vi "Program Setup.vi"(8 "error in (no error)":errorcluster, 10 "shutdown":refnum<user-event>, 11 "Modules":T8) -> (0 "error out":errorcluster)   [LabVIEW 2025]
uses:
  Controls/Sequencer/save icon.ctl
  Controls/transparent tab control.ctl
  Controls/refresh button 2.ctl
  Controls/tests tab control.ctl
  Controls/json cluster.ctl
  <vilib>/Handler Framework/CmdQueue/Enqueue Single.vi
  00f64e30-74e4-4e09-a3ad-345c80b98643.vi
  <vilib>/JDP Science/JSONtext/Variant to JSON Text.vi
  <vilib>/JDP Science/JSONtext/LVClass Serializer/JSONtext LVClass Serializer.lvclass
  <vilib>/Handler Framework/Handler Framework.lvlib
  <vilib>/JDP Science/JSONtext/JSONtext.lvlib
  aee85382-6405-4b67-82e5-8524274b1efe.vi
panel:
  in  "Tab Control":T1
  in  "Program":u16(ring) items=["AC-97", "EVI-79"]
  in  "Refresh":T2
  in  "Tab Control 3":T3
  out "Wear_in 2":T4={"V"=24.0, "I"=0.5, "Cycles"=50.0, "On_Time_ms"=100.0, "Off_Time_ms"=900.0}
  out "Drop_out 2":T5={"V"=24.0, "I"=0.5, "V_reduced"=4.0, "V_perturb"=0.01, "Plunger_Threshold"=0.01, "V_MIN"=1.0}
  out "CRT 2":cluster{"V":dbl, "I":dbl, "CRT_MAX_ms":dbl}={"V"=24.0, "I"=0.5, "CRT_MAX_ms"=100.0}
  out "Pull_in 2":T6={"V"=0.0, "I"=0.5, "V_increased"=9.0, "V_perturb"=0.01, "Plunger_Threshold"=0.01, "V_MAX"=13.0}
  out "Electrical_Properties 2":cluster{"V_max":dbl, "I_max":dbl}={"V_max"=24.0, "I_max"=0.5}
  out "ORT 2":cluster{"V":dbl, "I":dbl, "ORT_MAX_ms":dbl}={"V"=24.0, "I"=0.5, "ORT_MAX_ms"=100.0}
  in  "Program Name":string
  in  "Tab Control 2":T3
  in  "Wear_in":T4={"V"=24.0, "I"=0.5, "Cycles"=50.0, "On_Time_ms"=100.0, "Off_Time_ms"=900.0}
  in  "Drop_out":T5={"V"=24.0, "I"=0.5, "V_reduced"=4.0, "V_perturb"=0.01, "Plunger_Threshold"=0.01, "V_MIN"=1.0}
  in  "CRT":cluster{"V":dbl, "I":dbl, "CRT_MAX_ms":dbl}={"V"=24.0, "I"=0.5, "CRT_MAX_ms"=100.0}
  in  "Pull_in":T6={"V"=0.0, "I"=0.5, "V_increased"=9.0, "V_perturb"=0.01, "Plunger_Threshold"=0.01, "V_MAX"=13.0}
  in  "Electrical_Properties":cluster{"V_max":dbl, "I_max":dbl}={"V_max"=24.0, "I_max"=0.5}
  in  "ORT":cluster{"V":dbl, "I":dbl, "ORT_MAX_ms":dbl}={"V"=24.0, "I"=0.5, "ORT_MAX_ms"=100.0}
  in  "Save Program":T7
  # "Edit Programs"
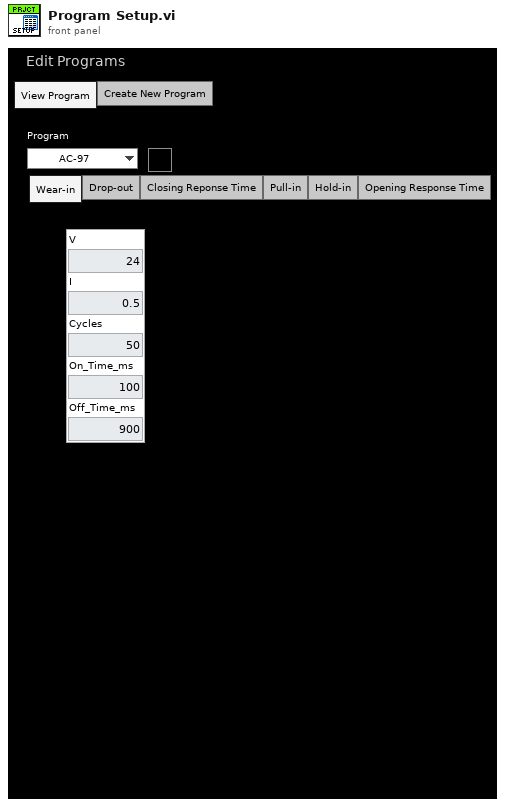
[diagram p1: front panel]
types:
  T1 = typedef "transparent tab control.ctl" = enum32{"View Program", "Create New Program"}
  T2 = typedef "refresh button 2.ctl" = bool
  T3 = typedef "tests tab control.ctl" = enum32{"Wear-in", "Drop-out", "Closing Reponse Time", "Pull-in", "Hold-in", "Opening Response Time"}
  T4 = cluster{"V":dbl, "I":dbl, "Cycles":dbl, "On_Time_ms":dbl, "Off_Time_ms":dbl}
  T5 = cluster{"V":dbl, "I":dbl, "V_reduced":dbl, "V_perturb":dbl, "Plunger_Threshold":dbl, "V_MIN":dbl}
  T6 = cluster{"V":dbl, "I":dbl, "V_increased":dbl, "V_perturb":dbl, "Plunger_Threshold":dbl, "V_MAX":dbl}
  T7 = typedef "save icon.ctl" = bool
  T8 = cluster{"Module IDs":i32[], "Module Names":string[]}
  T9 = enum16{"open", "replace", "create", "open or create", "replace or create", "replace or create with confirmation"}
  T10 = typedef "json cluster.ctl" = cluster{"Electrical_Properties":cluster{"V_max":dbl, "I_max":dbl}, "Wear_in":cluster{"V":dbl, "I":dbl, "Cycles":dbl, "On_Time_ms":dbl, "Off_Time_ms":dbl}, "Drop_out":cluster{"V":dbl, "I":dbl, "V_reduced":dbl, "V_perturb":dbl, "Plunger_Threshold":dbl, "V_MIN":dbl}, "ORT":cluster{"V":dbl, "I":dbl, "ORT_MAX_ms":dbl}, "CRT":cluster{"V":dbl, "I":dbl, "ORT_MAX_ms":dbl}, "Pull_in":cluster{"V":dbl, "I":dbl, "V_increased":dbl, "V_perturb":dbl, "Plunger_Threshold":dbl, "V_MAX":dbl}}
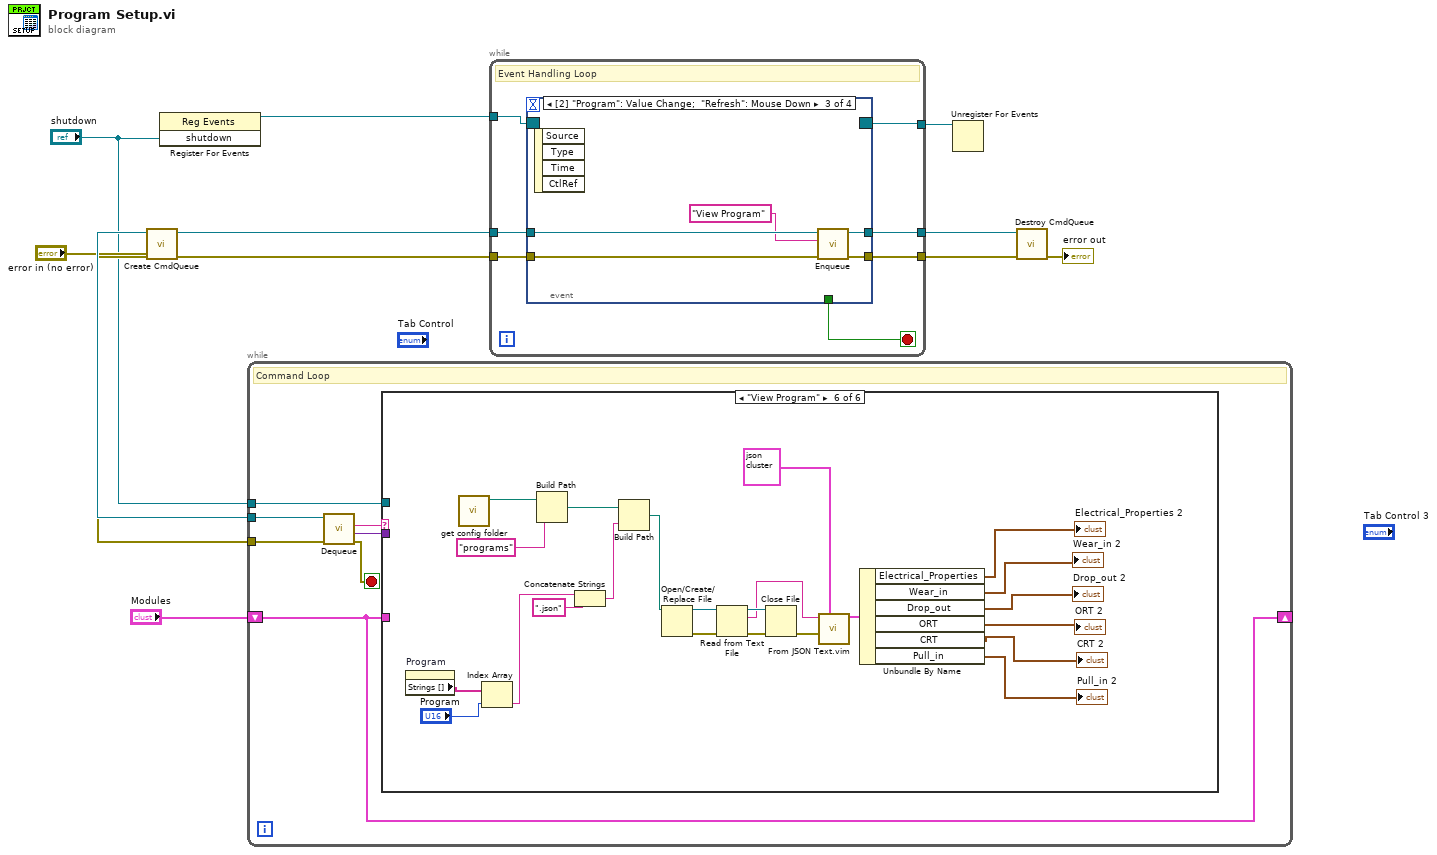
[diagram p0: block diagram]
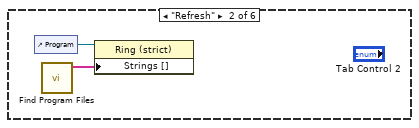
[diagram p3: hidden frame]
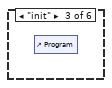
[diagram p4: hidden frame]
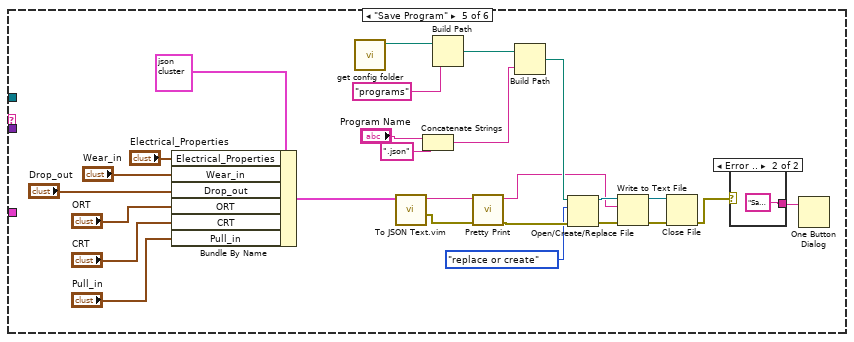
[diagram p6: hidden frame]
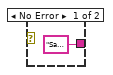
[diagram p7: hidden frame]
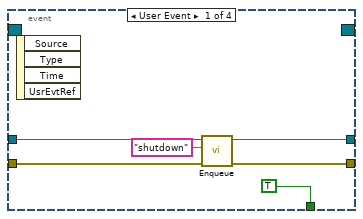
[diagram p8: hidden frame]
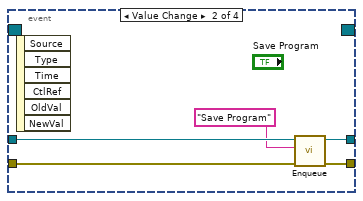
[diagram p9: hidden frame]
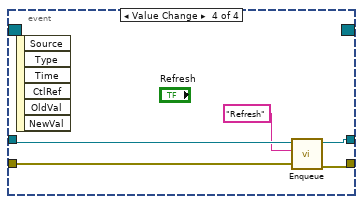
[diagram p10: hidden frame]
diagram:
  n1 = call <vilib>:"Create CmdQueue.vi"("error in (no error)"="error in (no error)") -> ("error out"=w7:errorcluster, "CmdQueue out"=w8:refnum<queue>)  [unwired: 9 in]
  n2 = register-events("shutdown") -> (reference out=w6:refnum<event-registration>)  [unwired: 2 in, 1 out]
  n3 = while {
    tunnel: w8 -> [w17]
    tunnel: w7 -> [w13]
    tunnel: "shutdown" -> [w12]
    shift-right: [w11] -> _
    shift-left: "Modules" -> [w11]
    stop <- w14 stop-if-true
    # "Command Loop"
    n4 = call <vilib>:"Dequeue.vi"("error in (no error)"=w13, "CmdQueue in"=w17) -> ("error out"=w14:errorcluster, "value"=w15:variant, "cmd"=w16:string)  [unwired: 5 in, 2 out]
    n5 = case shown="\"View Program\"" w16 {
      tunnel: w15 -> [_ _ _ _ _ _]
      tunnel: w12 -> [_ _ _ _ _ _]
      tunnel: w11 -> [_ _ _ _ _ _]
      frame "False", Default {
      }
      frame "Refresh" {
        n6 = control-ref of="Program"() -> (w19:refnum<vi>)
        n7 = call "Find Program Files.vi"() -> ("Array"=w18:string[])  [unwired: 10 in, 1 out]
        n8 = property class="Ring (strict)"(reference=w19, "Strings []"=w18) -> ()  [unwired: 1 in, 2 out]
      }
      frame "init" {
        n9 = control-ref of="Program"() -> ()  [unwired: 1 out]
      }
      frame "shutdown" {
      }
      frame "Save Program" {
        n10 = Bundle By Name(cluster=T10 {"Electrical_Properties"={"V_max"=24.0, "I_max"=0.5}, "Wear_in"={"V"=24.0, "I"=0.5, "Cycles"=0.5, "On_Time_ms"=0.5, "Off_Time_ms"=0.5}, "Drop_out"={"V"=24.0, "I"=0.5, "V_reduced"=4.0, "V_perturb"=0.01, "Plunger_Threshold"=0.01, "V_MIN"=1.0}, "ORT"={"V"=24.0, "I"=0.5, "ORT_MAX_ms"=100.0}, "CRT"={"V"=24.0, "I"=0.5, "ORT_MAX_ms"=100.0}, "Pull_in"={"V"=0.0, "I"=0.5, "V_increased"=9.0, "V_perturb"=0.01, "Plunger_Threshold"=0.01, "V_MAX"=1.0}} ("json cluster"), "Electrical_Properties"="Electrical_Properties", "Wear_in"="Wear_in", "Drop_out"="Drop_out", "ORT"="ORT", "CRT"="CRT", "Pull_in"="Pull_in") -> (w38:T10)
        n11 = call "get config folder.vi"() -> ("Config folder path"=w33:path)  [unwired: 11 in]
        n12 = call "To JSON Text.vim"("Anything"=w38) -> ("error out"=w36:errorcluster, "<JSON>"=w37:string)  [unwired: 9 in]
        n13 = Concatenate Strings("Program Name", ".json" ("string")) -> (w29:string)
        n14 = Build Path(base path=w33, name or relative path="programs") -> (appended path=w30:path)
        n15 = call <vilib>:"Pretty Print.vi"("error in (no error)"=w36, "JSON"=w37) -> ("error out"=w27:errorcluster, "<JSON>"=w25:string)  [unwired: 7 in, 1 out]
        n16 = Build Path(base path=w30, name or relative path=w29) -> (appended path=w28:path)
        n17 = Open/Create/Replace File(file path (use dialog)=w28, error in=w27, operation (0:open)=T9."replace or create") -> (refnum out=w35:refnum<file>, error out=w24:errorcluster)  [unwired: 3 in, 1 out]
        n18 = Write to Text File(file (use dialog)=w35, text=w25, error in=w24) -> (refnum out=w22:refnum<file>, error out=w23:errorcluster)  [unwired: 1 in, 1 out]
        n19 = Close File(refnum=w22, error in=w23) -> (error out=w21:errorcluster)  [unwired: 1 out]
        n20 = case shown="Error .." w21 {
          tunnel: ["Save succesful!" "Save failed.ave succesful!"] -> w20
          frame No Error {
          }
          frame Error {
          }
        }
        n21 = One Button Dialog(message=w20) -> ()  [unwired: 1 in, 1 out]
      }
      frame "View Program" {
        n22 = property on="Program" class="Ring (strict)"() -> ("Strings []"=w50:string[])  [unwired: 2 in, 2 out]
        n23 = call "get config folder.vi"() -> ("Config folder path"=w55:path)  [unwired: 11 in]
        n24 = Index Array(array=w50, index="Program") -> (element=w48:string)
        n25 = Build Path(base path=w55, name or relative path="programs") -> (appended path=w53:path)
        n26 = Concatenate Strings(w48, ".json" ("string")) -> (w52:string)
        n27 = Build Path(base path=w53, name or relative path=w52) -> (appended path=w51:path)
        n28 = Open/Create/Replace File(file path (use dialog)=w51) -> (refnum out=w70:refnum<file>, error out=w69:errorcluster)  [unwired: 5 in, 1 out]
        n29 = Read from Text File(file (use dialog)=w70, error in=w69) -> (refnum out=w67:refnum<file>, text=w64:string, error out=w68:errorcluster)  [unwired: 2 in, 1 out]
        n30 = Close File(refnum=w67, error in=w68) -> (error out=w66:errorcluster)  [unwired: 1 out]
        n31 = call "From JSON Text.vim"("Data Type and Default Value"=T10 {"Electrical_Properties"={"V_max"=24.0, "I_max"=0.5}, "Wear_in"={"V"=24.0, "I"=0.5, "Cycles"=0.5, "On_Time_ms"=0.5, "Off_Time_ms"=0.5}, "Drop_out"={"V"=24.0, "I"=0.5, "V_reduced"=4.0, "V_perturb"=0.01, "Plunger_Threshold"=0.01, "V_MIN"=1.0}, "ORT"={"V"=24.0, "I"=0.5, "ORT_MAX_ms"=100.0}, "CRT"={"V"=24.0, "I"=0.5, "ORT_MAX_ms"=100.0}, "Pull_in"={"V"=0.0, "I"=0.5, "V_increased"=9.0, "V_perturb"=0.01, "Plunger_Threshold"=0.01, "V_MAX"=1.0}} ("json cluster"), "error in (no error)"=w66, "JSON"=w64) -> ("Data out"=w63:T10)  [unwired: 7 in, 1 out]
        n32 = Unbundle By Name(w63) -> ("Electrical_Properties"=→"Electrical_Properties 2":cluster{"V_max":dbl, "I_max":dbl}, "Wear_in"=→"Wear_in 2":T4, "Drop_out"=→"Drop_out 2":T5, "ORT"=→"ORT 2":cluster{"V":dbl, "I":dbl, "ORT_MAX_ms":dbl}, "CRT"=→"CRT 2":cluster{"V":dbl, "I":dbl, "ORT_MAX_ms":dbl}, "Pull_in"=→"Pull_in 2":T6)
      }
    }
  }
  n33 = while {
    tunnel: w8 -> [w77]
    tunnel: [w76] -> w10
    tunnel: w7 -> [w75]
    tunnel: [w74] -> w9
    tunnel: w6 -> [w72]
    tunnel: [w71] -> w5
    stop <- w73 stop-if-true
    # "Event Handling Loop"
    n34 = event shown="[2] \"Program\": Value Change;  \"Refresh\": Mouse Down" {
      selector: w72 -> [_ _ _ _]
      dyn-events: [_ _ _ _] -> w71
      timeout: _ -> [_ _ _ _]
      tunnel: w77 -> [w83 w86 w91 w96]
      tunnel: [w82 w87 w92 w97] -> w76
      tunnel: w75 -> [w81 w85 w90 w95]
      tunnel: [w80 w88 w93 w98] -> w74
      tunnel: [TRUE ("Discard?") _ _ _] -> w73
      event User Event {
        n35 = event-data() -> ()  [unwired: 1 in, 4 out]
        n36 = call-poly <vilib>:"Enqueue.vi"("error in (no error)"=w81, "Command"="shutdown", "CmdQueue in"=w83) -> ("error out"=w80:errorcluster, "CmdQueue out"=w82:refnum<queue>)  [unwired: 7 in]
      }
      event Value Change {
        n37 = event-data() -> ()  [unwired: 1 in, 6 out]
        n38 = call-poly <vilib>:"Enqueue.vi"("error in (no error)"=w85, "Command"="Save Program", "CmdQueue in"=w86) -> ("error out"=w88:errorcluster, "CmdQueue out"=w87:refnum<queue>)  [unwired: 7 in]
      }
      event "Program": Value Change; Mouse Down {
        n39 = event-data() -> ()  [unwired: 1 in, 4 out]
        n40 = call-poly <vilib>:"Enqueue.vi"("error in (no error)"=w90, "Command"="View Program", "CmdQueue in"=w91) -> ("error out"=w93:errorcluster, "CmdQueue out"=w92:refnum<queue>)  [unwired: 7 in]
      }
      event Value Change {
        n41 = event-data() -> ()  [unwired: 1 in, 6 out]
        n42 = call-poly <vilib>:"Enqueue.vi"("error in (no error)"=w95, "Command"="Refresh", "CmdQueue in"=w96) -> ("error out"=w98:errorcluster, "CmdQueue out"=w97:refnum<queue>)  [unwired: 7 in]
      }
    }
  }
  n43 = Unregister For Events(event registration refnum=w5) -> ()  [unwired: 1 in, 1 out]
  n44 = call <vilib>:"Destroy CmdQueue.vi"("error in (no error)"=w9, "CmdQueue in"=w10) -> ("error out"=→"error out":errorcluster)  [unwired: 9 in]
